vi "Get Register Address.vi"(8 "error in (no error)":errorcluster, 11 "RFFE Command in":refnum<class "RFFE Command.lvclass">) -> (0 "error out":errorcluster, 2 "Register Address":T1 format="%02x", 3 "RFFE Command out":refnum<class "RFFE Command.lvclass">)   [LabVIEW 2018, in "MIPI RFFE API.lvlib" / "RFFE Command.lvclass"]
uses:
  RFFE Command.lvclass
  Register Address.ctl
  RFFE Command.lvclass/RFFE Command.ctl
  MIPI RFFE API.lvlib
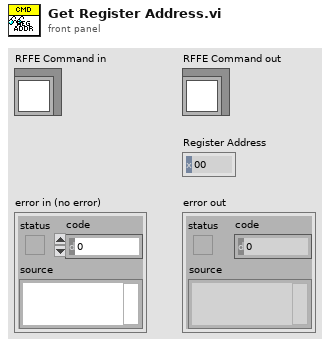
[diagram p1: front panel]
types:
  T1 = typedef "MIPI RFFE API.lvlib/Register Address.ctl" = u16
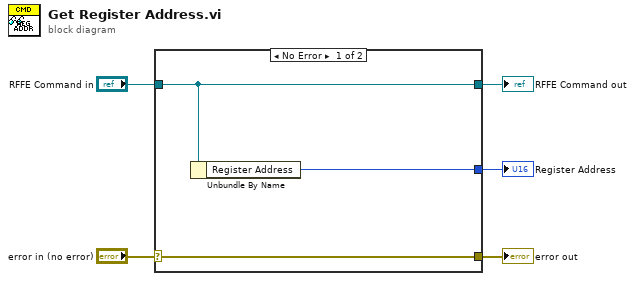
[diagram p0: block diagram]
diagram:
  n1 = case shown="No Error" "error in (no error)" {
    selector: "error in (no error)" -> [w8 w9]
    tunnel: [w8 w9] -> w4
    tunnel: [w7 w10] -> w2
    tunnel: "RFFE Command in" -> [w7 w10]
    tunnel: [w6 _] -> w1
    frame No Error {
      n2 = Unbundle By Name(w7) -> ("Register Address"=w6:T1)
    }
    frame Error {
    }
  }
  "error out" <- w4
  "RFFE Command out" <- w2
  "Register Address" <- w1
